vi "List-All-Label's.vi"(8 "error in (no error)":errorcluster, 11 "Quick-GUI-Update in":refnum<class "Quick-GUI-Update.lvclass">) -> (0 "error out":errorcluster, 1 "Label's List":string[][](array[string]), 3 "Quick-GUI-Update out":refnum<class "Quick-GUI-Update.lvclass">)   [LabVIEW 2020, in "Easy GUI Operation.lvlib" / "Quick-GUI-Update.lvclass"]
uses:
  Quick-GUI-Update.lvclass
  Quick-GUI-Update.lvclass/Quick-GUI-Update.ctl
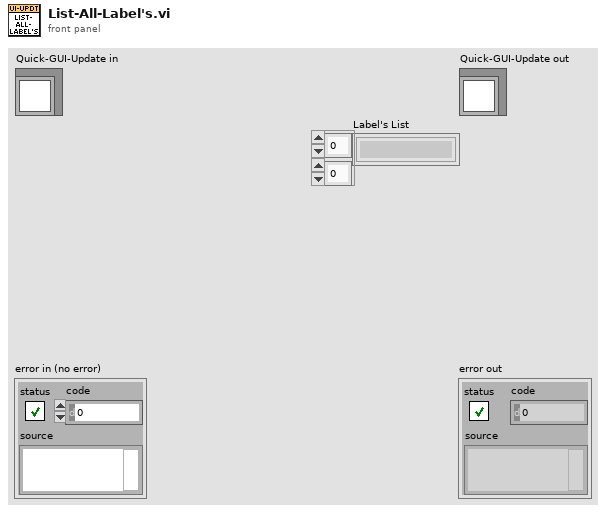
[diagram p1: front panel]
types:
  T1 = map{string, set{cluster{"Ctrl-Ref":refnum<vi>, "Ctrl Index":i32, "Class-Name":string, "Class ID":u32}}}
  T2 = set{cluster{"Ctrl-Ref":refnum<vi>, "Ctrl Index":i32, "Class-Name":string, "Class ID":u32}}
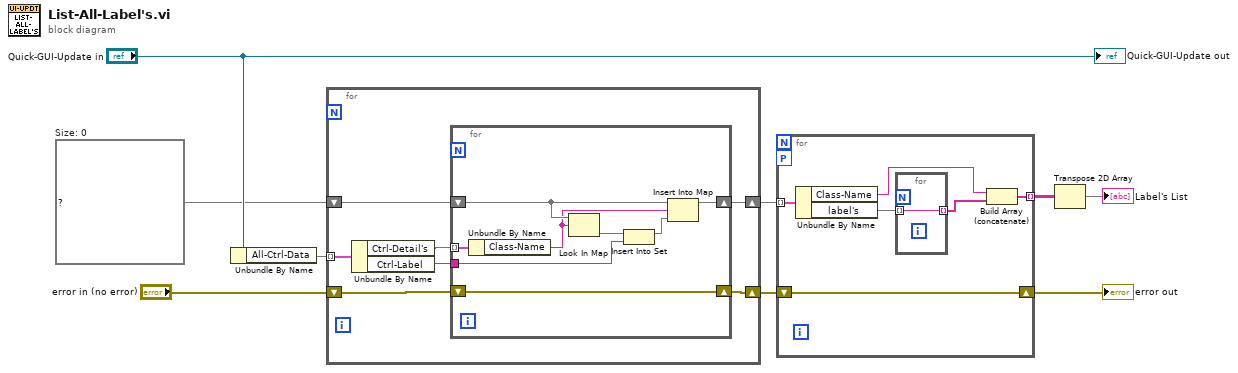
[diagram p0: block diagram]
diagram:
  w6 = map{string, set{string}} {}  # Size: 0
  n1 = Unbundle By Name("Quick-GUI-Update in") -> ("All-Ctrl-Data"=w1:T1)
  n2 = for {
    shift-right: [w13] -> w3
    shift-left: w6 -> [w15]
    shift-right: [w12] -> w2
    shift-left: "error in (no error)" -> [w11]
    tunnel: w1 -> [w16] mode=indexing
    n3 = Unbundle By Name(w16) -> ("Ctrl-Detail's"=w10:T2, "Ctrl-Label"=w14:string)
    n4 = for {
      tunnel: w10 -> [w24] mode=indexing
      shift-right: [w19] -> w13
      shift-left: w15 -> [w21]
      tunnel: w14 -> [w22]
      shift-right: [w17] -> w12
      shift-left: w11 -> [w17]
      n5 = Unbundle By Name(w24) -> ("Class-Name"=w20:string)
      n6 = Look In Map(map=w21, key=w20) -> (value=w23:set{string})  [unwired: 1 in, 1 out]
      n7 = Insert Into Set(10:w22, 11:w23) -> (3:w18:set{string})  [unwired: 1 out]
      n8 = Insert Into Map(map in=w21, key=w20, value=w18) -> (map out=w19:map{string, set{string}})  [unwired: 2 out]
    }
  }
  n9 = for {
    tunnel: w3 -> [w30] mode=indexing
    tunnel: [w26] -> w5 mode=indexing
    shift-right: [w25] -> w8
    shift-left: w2 -> [w25]
    workers-P: _ -> [_]
    n10 = Unbundle By Name(w30) -> ("Class-Name"=w27:string, "label's"=w29:set{string})
    n11 = for {
      tunnel: w29 -> [w31] mode=indexing
      tunnel: [w31] -> w28 mode=indexing
    }
    n12 = Build Array (concatenate)(w27, w28) -> (w26:string[])
  }
  "error out" <- w8
  n13 = Transpose 2D Array(2D array=w5) -> (transposed array=→"Label's List":string[][])
  "Quick-GUI-Update out" <- "Quick-GUI-Update in"
